vi "DrawInvaders.vi"(8 "error in":errorcluster, 10 "InitCluster_IN":T1, 11 "InvaderArray":bool[][](array[boolean])=[[TRUE, TRUE, TRUE, TRUE, TRUE, TRUE, TRUE, TRUE, TRUE, TRUE], [TRUE, TRUE, TRUE, TRUE, TRUE, TRUE, TRUE, TRUE, TRUE, TRUE], [TRUE, TRUE, TRUE, TRUE, TRUE, TRUE, TRUE, TRUE, TRUE, TRUE], [TRUE, TRUE, TRUE, TRUE, TRUE, TRUE, TRUE, TRUE, TRUE, TRUE], [TRUE, TRUE, TRUE, TRUE, TRUE, TRUE, TRUE, TRUE, TRUE, TRUE]]) -> (0 "error out":errorcluster, 2 "InitCluster_OUT":T1, 3 "InvaderPosArray":T7(array[cluster]))   [LabVIEW 2019]
uses:
  InitCluster.ctl
  CharacterCluster.ctl
  <vilib>/picture/picture.llb/imagedata.ctl
  ShotInitCluster.ctl
  <vilib>/Utility/miscctls.llb/LVPositionTypeDef.ctl
  <vilib>/Utility/miscctls.llb/LVBoundsTypeDef.ctl
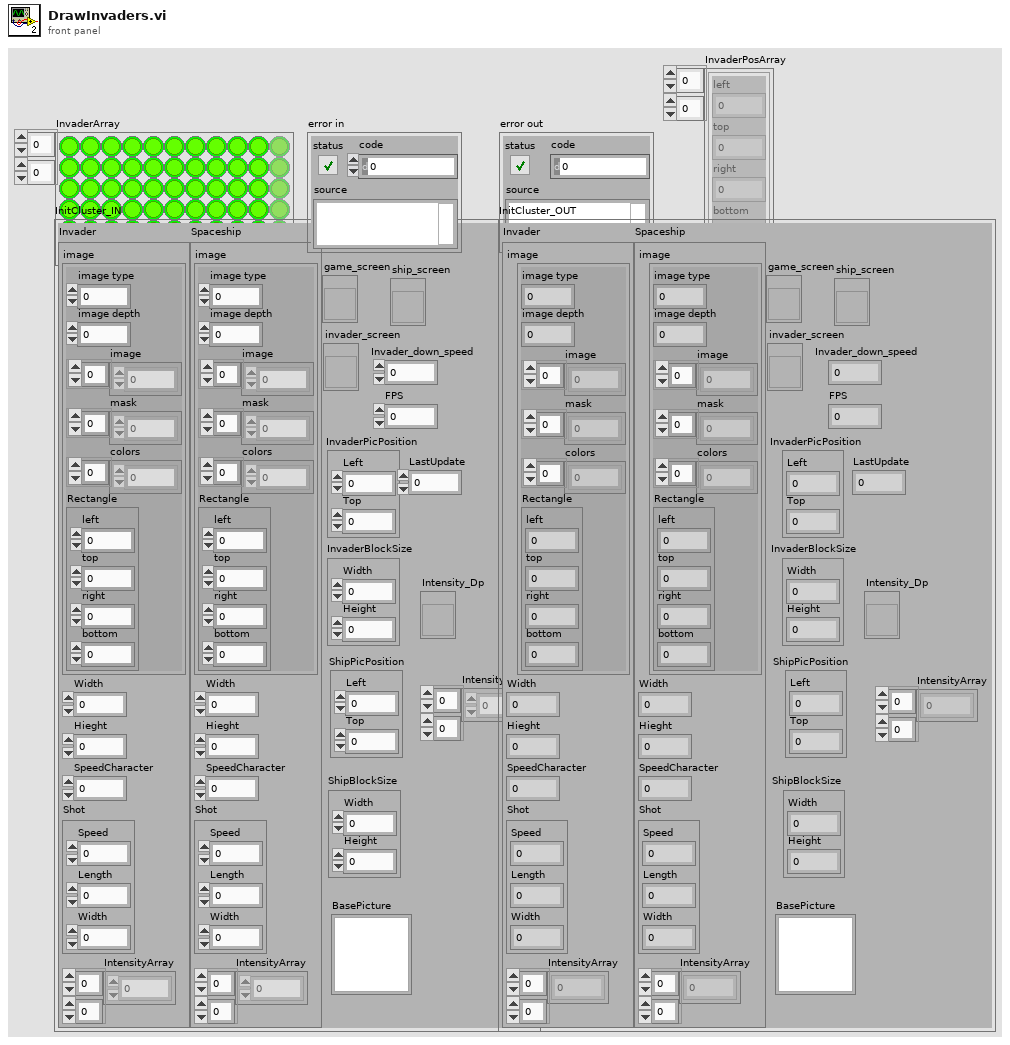
[diagram p1: front panel]
types:
  T1 = typedef "InitCluster.ctl" = cluster{"Invader":T2, "Spaceship":T2, "game_screen":refnum<vi>, "BasePicture":picture, "invader_screen":refnum<vi>, "InvaderPicPosition":T5, "Invader_down_speed":i16, "FPS":u16, "InvaderBlockSize":T6, "ship_screen":refnum<vi>, "ShipBlockSize":T6, "ShipPicPosition":T5, "LastUpdate":u32, "Intensity_Dp":refnum<vi>, "IntensityArray":u8[][]}
  T2 = typedef "CharacterCluster.ctl" = cluster{"image":T3, "Width":u32, "Hieght":u32, "SpeedCharacter":u32, "Shot":T4, "IntensityArray":u8[][]}
  T3 = typedef "imagedata.ctl" = cluster{"image type":i32, "image depth":i32, "image":u8[], "mask":u8[], "colors":u32[], "Rectangle":cluster{"left":i16, "top":i16, "right":i16, "bottom":i16}}
  T4 = typedef "ShotInitCluster.ctl" = cluster{"Speed":u32, "Length":u32, "Width":u32}
  T5 = typedef "LVPositionTypeDef.ctl" = cluster{"Left":i32, "Top":i32}
  T6 = typedef "LVBoundsTypeDef.ctl" = cluster{"Width":u32, "Height":u32}
  T7 = cluster{"left":i16, "top":i16, "right":i16, "bottom":i16}[][]
  T8 = cluster{"left":i16, "top":i16, "right":i16, "bottom":i16}
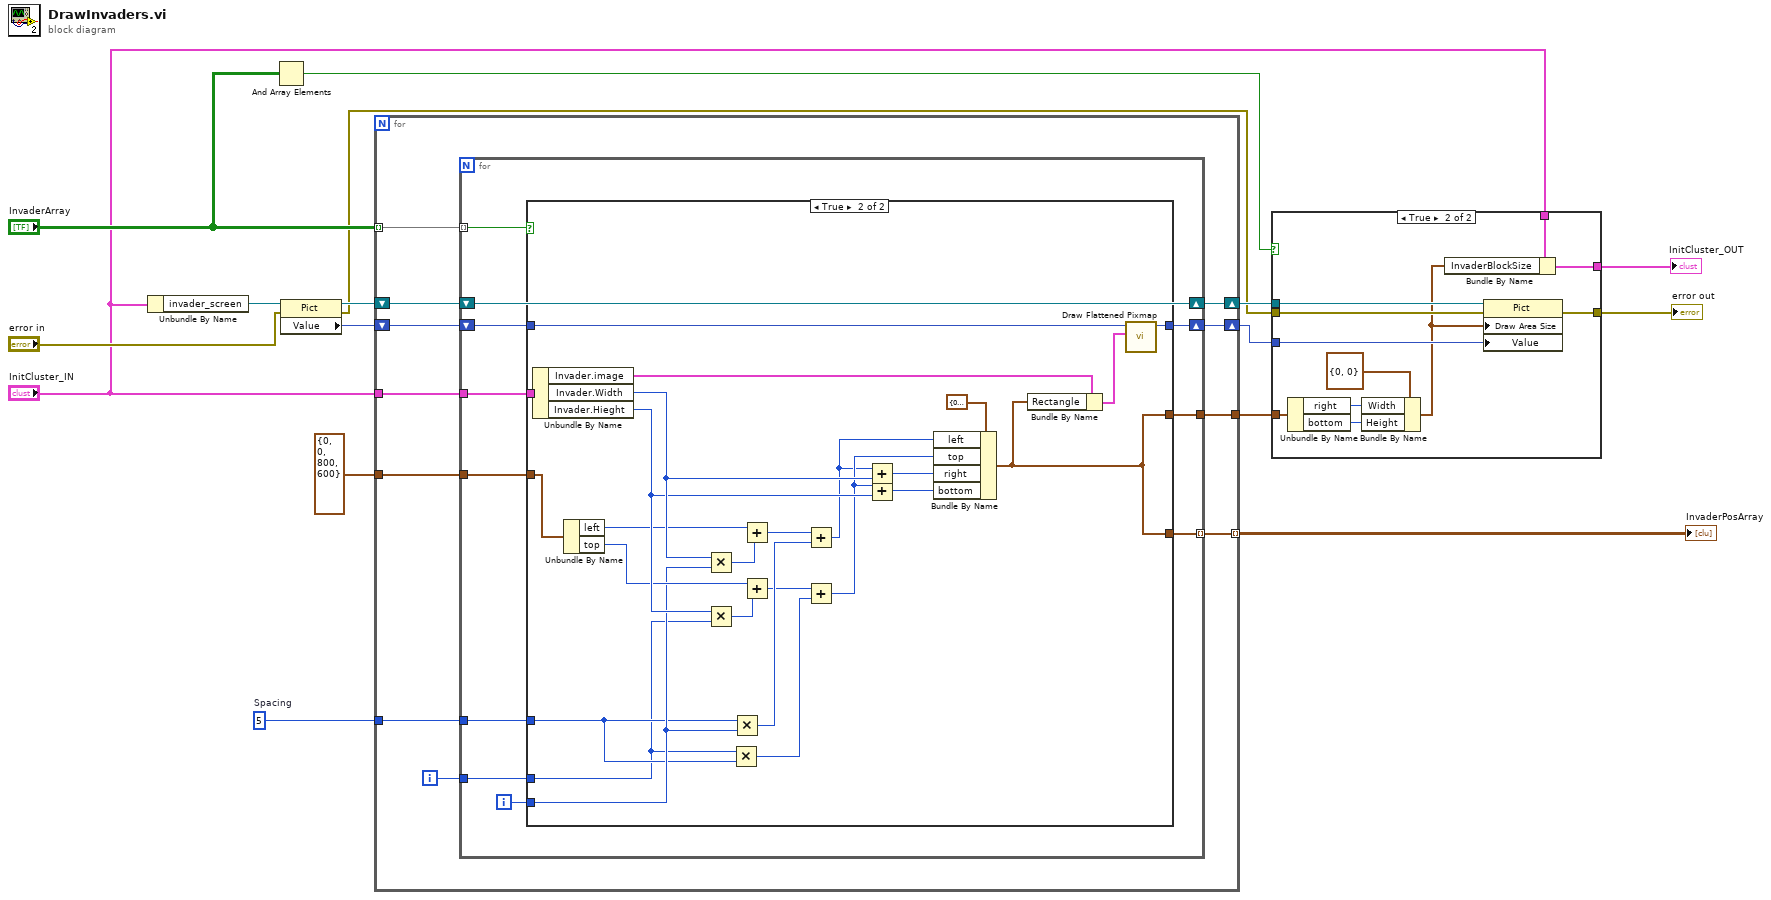
[diagram p0: block diagram]
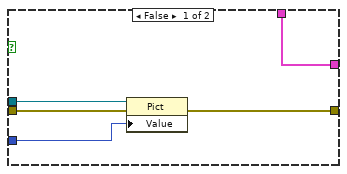
[diagram p2: hidden frame]
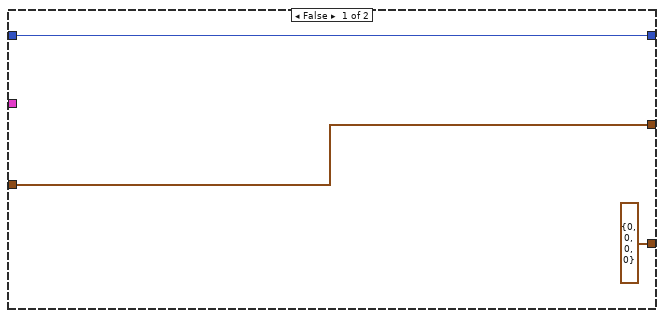
[diagram p3: hidden frame]
diagram:
  w11 = 5  # Spacing
  n1 = Unbundle By Name("InitCluster_IN") -> ("invader_screen"=w16:refnum<vi>)
  n2 = And Array Elements(Boolean array="InvaderArray") -> (logical AND=w1:bool)
  n3 = property class="Pict"(reference=w16, error in="error in") -> (reference out=w13:refnum<vi>, error out=w4:errorcluster, "Value"=w15:picture)
  n4 = for {
    tunnel: "InvaderArray" -> [w27] mode=indexing
    tunnel: T8 {"left"=0, "top"=0, "right"=800, "bottom"=600} ("TopLeftCorner") -> [w26]
    shift-right: [w22] -> w3
    shift-left: w15 -> [w25]
    tunnel: "InitCluster_IN" -> [w24]
    shift-right: [w20] -> w5
    shift-left: w13 -> [w21]
    tunnel: w11 -> [w19]
    tunnel: [w18] -> w10 mode=indexing
    tunnel: [w17] -> w8
    i -> [w23]
    n5 = for {
      tunnel: w27 -> [w33] mode=indexing
      tunnel: w26 -> [w32]
      shift-right: [w35] -> w22
      shift-left: w25 -> [w38]
      tunnel: w24 -> [w37]
      tunnel: w23 -> [w30]
      shift-right: [w34] -> w20
      shift-left: w21 -> [w34]
      tunnel: w19 -> [w31]
      tunnel: [w29] -> w18 mode=indexing
      tunnel: [w28] -> w17
      i -> [w36]
      n6 = case shown="True" w33 {
        tunnel: w38 -> [w41 w66]
        tunnel: w37 -> [_ w65]
        tunnel: w36 -> [_ w52]
        tunnel: [w41 w60] -> w35
        tunnel: w32 -> [w39 w59]
        tunnel: w31 -> [_ w50]
        tunnel: w30 -> [_ w46]
        tunnel: [T8 {"left"=0, "top"=0, "right"=0, "bottom"=0} ("Rectangle") w42] -> w29
        tunnel: [w39 w42] -> w28
        frame False {
        }
        frame True {
          n7 = Unbundle By Name(w65) -> ("Invader.image"=w44:T3, "Invader.Width"=w64:u32, "Invader.Hieght"=w63:u32)
          n8 = Unbundle By Name(w59) -> ("left"=w57:i16, "top"=w55:i16)
          n9 = Multiply(x=w64, y=w52) -> (x*y=w58:u32)
          n10 = Multiply(x=w63, y=w46) -> (x*y=w56:u32)
          n11 = Multiply(x=w46, y=w50) -> (x*y=w49:i32)
          n12 = Multiply(x=w50, y=w52) -> (x*y=w51:i32)
          n13 = Add(x=w57, y=w58) -> (x+y=w54:u32)
          n14 = Add(x=w55, y=w56) -> (x+y=w47:u32)
          n15 = Add(x=w54, y=w51) -> (x+y=w48:u32)
          n16 = Add(x=w47, y=w49) -> (x+y=w53:u32)
          n17 = Add(x=w48, y=w64) -> (x+y=w62:u32)
          n18 = Add(x=w53, y=w63) -> (x+y=w61:u32)
          n19 = Bundle By Name(cluster=T8 {"left"=0, "top"=0, "right"=0, "bottom"=0} ("Rectangle"), "left"=w48, "top"=w53, "right"=w62, "bottom"=w61) -> (w42:T8)
          n20 = Bundle By Name(cluster=w44, "Rectangle"=w42) -> (w43:T3)
          n21 = call <vilib>:"Draw Flattened Pixmap.vi"("image data"=w43, "picture"=w66) -> ("new picture"=w60:picture)  [unwired: 7 in]
        }
      }
    }
  }
  "InvaderPosArray" <- w10
  n22 = case shown="True" w1 {
    tunnel: w8 -> [_ w82]
    tunnel: "InitCluster_IN" -> [w71 w81]
    tunnel: [w71 w80] -> w6
    tunnel: w5 -> [w70 w79]
    tunnel: w4 -> [w69 w78]
    tunnel: w3 -> [w68 w77]
    tunnel: [w67 w76] -> w2
    frame False {
      n23 = property class="Pict"(reference=w70, error in=w69, "Value"=w68) -> (error out=w67:errorcluster)  [unwired: 1 out]
    }
    frame True {
      n24 = Unbundle By Name(w82) -> ("right"=w74:i16, "bottom"=w75:i16)
      n25 = Bundle By Name(cluster=T6 {"Width"=0, "Height"=0} ("Draw Area Size"), "Width"=w74, "Height"=w75) -> (w72:T6)
      n26 = Bundle By Name(cluster=w81, "InvaderBlockSize"=w72) -> (w80:T1)
      n27 = property class="Pict"(reference=w79, error in=w78, "Draw Area Size"=w72, "Value"=w77) -> (error out=w76:errorcluster)  [unwired: 1 out]
    }
  }
  "error out" <- w2
  "InitCluster_OUT" <- w6
